vi "Associate Instruments to Paths.vi"(0 "SG Path Group in":refnum<class "SG Path Group.lvclass">, 5 "TSM Context":T1, 11 "error in":errorcluster) -> (4 "SG Path Group out":refnum<class "SG Path Group.lvclass">, 15 "error out":errorcluster)   [LabVIEW 2023, in "RFFixtureCharact.RMM.lvlib" / "SG Path Group.lvclass"]
uses:
  SG Path Group.lvclass
  C:/rfcal/AuxTools/STSRFFixtureCharactUtility/Source/Code Modules/Common/Base Classes/Path Group/Path Group.lvclass
  <vilib>/NI_TestStand_SemiconductorModule/NI_TestStand_Semiconductor_Module.lvlibp/PinMap/General/SemiconductorModuleContext.ctl
  Public/Base Classes/Scalar/SG Abstract Path/SG Abstract Path.lvclass
  Public/Charact Result Accessor/Scalar/Scalar Charact Result Accessor.lvclass
  C:/rfcal/AuxTools/STSRFFixtureCharactUtility/Source/Code Modules/Fixture/RMM/Charact Result Accessor/Base/Charact Result Accessor.lvclass
  C:/rfcal/AuxTools/STSRFFixtureCharactUtility/Source/Code Modules/Common/Result Accessor/Result Accessor.lvclass
  Public/Base Classes/Scalar/SG Path/SG Path.lvclass
  C:/rfcal/AuxTools/STSRFFixtureCharactUtility/Source/Code Modules/Common/Base Classes/Path/Path.lvclass
  C:/rfcal/AuxTools/STSRFFixtureCharactUtility/Source/Code Modules/Fixture/Public/Base Classes/Scalar/Scalar Path/Scalar Path.lvclass
  C:/rfcal/AuxTools/STSRFFixtureCharactUtility/Source/Code Modules/Fixture/Public/Base Classes/Scalar/SG Abstract Path/SG Abstract Path.lvclass
  Common/Base Classes/Path/Path.lvclass/Path.ctl
  Common/Base Classes/Path/Properties/Read Interval.vi
  <vilib>/NI_TestStand_SemiconductorModule/NI_TestStand_Semiconductor_Module.lvlibp/PinMap/RF/RFSG/PinToNIRFSGSession.vi
  Common/Base Classes/Path/Path.lvclass
  SG Path Group.lvclass/SG Path Group.ctl
  <vilib>/NI_TestStand_SemiconductorModule/NI_TestStand_Semiconductor_Module.lvlibp
  Common/Base Classes/Path Group/Path Group.lvclass
  <vilib>/addons/_RFCalAndCharactDatabase/NI_RFCalAndCharact_Database_API.lvlibp/Characterization/Characterization.lvlib
  Instruments/Power Meter/Power Meter Factory/Power Meter Factory.lvclass
  Common/RFCalAndFixtureCharact.Common.lvlib
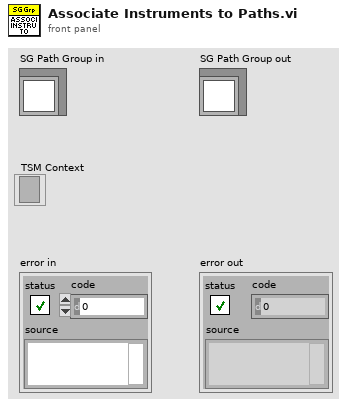
[diagram p1: front panel]
types:
  T1 = typedef "NI_TestStand_Semiconductor_Module.lvlibp/SemiconductorModuleContext.ctl" = refnum<k7>
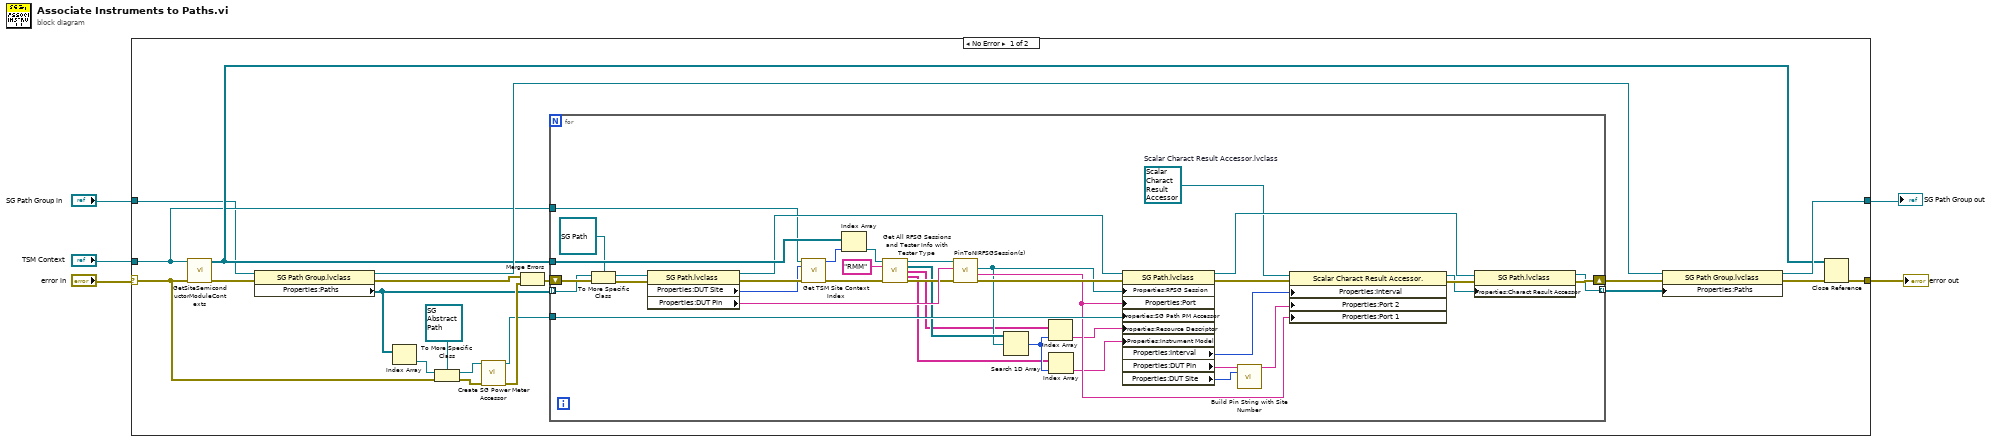
[diagram p0: block diagram]
diagram:
  n1 = case shown="No Error" "error in" {
    selector: "error in" -> [w9 w65]
    tunnel: "TSM Context" -> [w17 _]
    tunnel: "SG Path Group in" -> [w11 w64]
    tunnel: [w19 w65] -> w2
    tunnel: [w20 w64] -> w1
    frame No Error {
      n2 = call <vilib>:"GetSiteSemiconductorModuleContexts.vi"("error in (no error)"=w9, "Semiconductor Module Context"=w17) -> ("error out"=w24:errorcluster, "Site Semiconductor Module Contexts"=w18:T1[])  [unwired: 8 in]
      n3 = property class="SG Path Group.lvclass"(reference=w11, error in=w24) -> (reference out=w22:refnum<class "SG Path Group.lvclass">, error out=w15:errorcluster, "Properties:Paths"=w12:refnum<class "Path.lvclass">[])
      n4 = Index Array(array=w12) -> (element=w7:refnum<class "Path.lvclass">)  [unwired: 1 in]
      n5 = To More Specific Class(target class=refnum<class "SG Abstract Path.lvclass"> refnum ("RFFixtureCharact.Common.lvlib:SG Path.lvclass"), reference=w7, error in=w9) -> (specific class reference=w6:refnum<class "SG Abstract Path.lvclass">, error out=w10:errorcluster)
      n6 = call "Create SG Power Meter Accessor.vi"("SG Path"=w6, "error in"=w10) -> ("SG Path PM Accessor out"=w13:refnum<class "SG Path PM Accessor Base.lvclass">, "error out"=w14:errorcluster)  [unwired: 12 in]
      n7 = Merge Errors(w15, w14) -> (w16:errorcluster)
      n8 = for {
        tunnel: w18 -> [w63]
        tunnel: w12 -> [w43] mode=indexing
        shift-right: [w52] -> w25
        shift-left: w16 -> [w46]
        tunnel: [w50] -> w21 mode=indexing
        tunnel: w17 -> [w60]
        tunnel: w13 -> [w55]
        w26 = refnum<class "Scalar Charact Result Accessor.lvclass"> refnum  # Scalar Charact Result Accessor.lvclass
        n9 = To More Specific Class(target class=refnum<class "SG Path.lvclass"> refnum ("SG Path"), reference=w43, error in=w46) -> (specific class reference=w44:refnum<class "SG Path.lvclass">, error out=w45:errorcluster)
        n10 = property class="SG Path.lvclass"(reference=w44, error in=w45) -> (reference out=w62:refnum<class "SG Path.lvclass">, error out=w61:errorcluster, "Properties:DUT Site"=w59:i32, "Properties:DUT Pin"=w56:string)
        n11 = call "Get TSM Site Context Index.vi"("Semiconductor Module Context"=w60, "Site Number"=w59, "error in (no error)"=w61) -> ("index of Site TSM Context"=w58:i32, "error out"=w40:errorcluster)  [unwired: 11 in]
        n12 = Index Array(array=w63, index=w58) -> (element=w37:T1)
        n13 = call "Get All RFSG Sessions and Tester Info with Tester Type.vi"("TSM Context In"=w37, "Tester Type"="RMM", "error in"=w40) -> ("TSM Context Out"=w38:T1, "RFSG Sessions"=w36:refnum<k15>[], "Resource Descriptors"=w33:string[], "Instrument Models"=w32:string[], "error out"=w39:errorcluster)  [unwired: 8 in]
        n14 = call-poly <vilib>:"PinToNIRFSGSession(s).vi"("error in (no error)"=w39, "Pin"=w56, "Semiconductor Module Context"=w38) -> ("error out"=w57:errorcluster, "Port"=w54:string, "Instrument Session"=w34:refnum<k15>)  [unwired: 4 in, 2 out]
        n15 = Search 1D Array(1D array=w36, element=w34) -> (index of element=w41:i32)  [unwired: 1 in]
        n16 = Index Array(array=w33, index=w41) -> (element=w31:string)
        n17 = Index Array(array=w32, index=w41) -> (element=w30:string)
        n18 = property class="SG Path.lvclass"(reference=w62, error in=w57, "Properties:RFSG Session"=w34, "Properties:Port"=w54, "Properties:SG Path PM Accessor"=w55, "Properties:Resource Descriptor"=w31, "Properties:Instrument Model"=w30) -> (reference out=w51:refnum<class "SG Path.lvclass">, error out=w27:errorcluster, "Properties:Interval"=w28:i32, "Properties:DUT Pin"=w48:string, "Properties:DUT Site"=w47:i32)
        n19 = call <vilib>:"Build Pin String with Site Number.vi"("Pin Name"=w48, "Site Number"=w47) -> ("Pin String"=w29:string)  [unwired: 13 in]
        n20 = property class="Scalar Charact Result Accessor."(reference=w26, error in=w27, "Properties:Interval"=w28, "Properties:Port 2"=w29, "Properties:Port 1"=w54) -> (reference out=w49:refnum<class "Scalar Charact Result Accessor.lvclass">, error out=w53:errorcluster)
        n21 = property class="SG Path.lvclass"(reference=w51, error in=w53, "Properties:Charact Result Accessor"=w49) -> (reference out=w50:refnum<class "SG Path.lvclass">, error out=w52:errorcluster)
      }
      n22 = property class="SG Path Group.lvclass"(reference=w22, error in=w25, "Properties:Paths"=w21) -> (reference out=w20:refnum<class "SG Path Group.lvclass">, error out=w23:errorcluster)
      n23 = Close Reference(reference=w18, error in (no error)=w23) -> (error out=w19:errorcluster)
    }
    frame Error {
    }
  }
  "error out" <- w2
  "SG Path Group out" <- w1
